vi "Simulation Driver.vi"() -> ()   [LabVIEW 2016]
uses:
  subVIs/Global Variables.vi
panel:
  in  "Data Queue":refnum<queue>
  in  "Background Image":refnum<vi>
  in  "Inkscape File (.svg)":refnum<vi>
  in  "Run":refnum<vi>
  in  "Abort":refnum<vi>
  in  "Lithography Data":T1(array[cluster])
  # "Usually these controls will be hidden\nand settings will be displayed here."
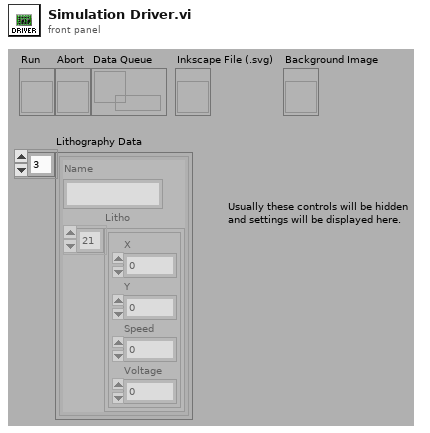
[diagram p1: front panel]
types:
  T1 = cluster{"Name":string, "Litho":cluster{"X":dbl, "Y":dbl, "Speed":dbl, "Voltage":dbl}[]}[]
  T2 = cluster{"X Offset (µm)":dbl, "Y Offset (µm)":dbl}
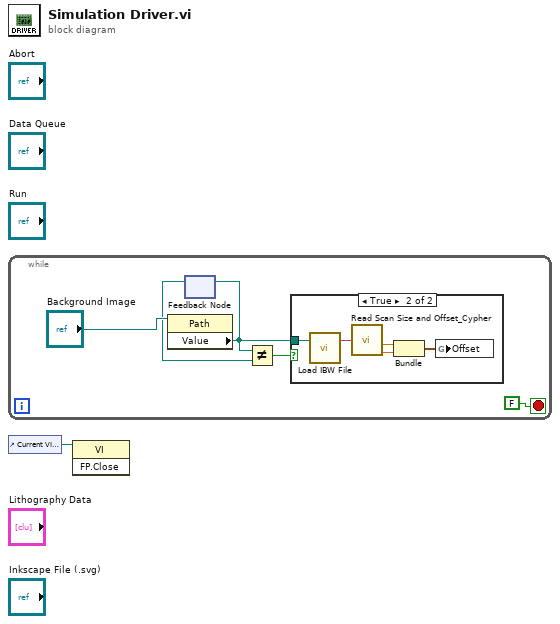
[diagram p0: block diagram]
diagram:
  n1 = while {
    stop <- FALSE stop-if-true
    n2 = property class="Path"(reference="Background Image") -> ("Value"=w4:path)  [unwired: 1 in, 2 out]
    n3 = feedback #1() -> (w2:path)  [unwired: 1 in]
    n4 = feedback-in #1(w4) -> ()
    n5 = Not Equal?(x=w4, y=w2) -> (x != y?=w3:bool)
    n6 = case shown="True" w3 {
      tunnel: w4 -> [_ w8]
      frame False {
      }
      frame True {
        n7 = call "Load IBW File.vi"("file path (dialog if empty)"=w8) -> ("Wave Note"=w7:string)  [unwired: 1 in, 1 out]
        n8 = call "Read Scan Size and Offset_Cypher.vi"("Read in the string file"=w7) -> ("X Offset (µm)"=w11:dbl, "Y Offset (µm)"=w10:dbl)  [unwired: 4 in, 2 out]
        n9 = Bundle("X Offset (µm)"=w11, "Y Offset (µm)"=w10) -> (w9:T2)  [unwired: 1 in]
        n10 = global write "Global Variables.vi" "Offset"(w9) -> ()
      }
    }
  }
  n11 = control-ref of="Current VI Reference"() -> (w1:refnum<vi>)
  n12 = invoke class="VI" method="FP.Close"(reference=w1) -> ()  [unwired: 2 in, 3 out]
